vi "Load Production his.vi"(8 "error in (no error)":errorcluster, 9 "Error info (end)":timestamp=timestamp(3727674196.4539065 s since 1904-01-01) format="%<%Y/%m/%d>T", 10 "Error info (start)":timestamp=timestamp(3727674196.4539065 s since 1904-01-01) format="%<%Y/%m/%d>T", 11 "DBlink":string="Driver={ODBC Driver 17 for SQL Server};Server=localhost\\SQLEXPRESS;Database=YDXB01;UID=labview;PWD=123456789") -> (0 "error out":errorcluster, 1 "production_report":T1(array[cluster])=[{"id"=13, "time_supply"="2022/2/14 ¤U¤È 06:05:43", "time_spout"="", "product_num"="F509", "barcode"="400010509", "box"="B", "quality"="NG", "section_time"=0, "total_time"=0}, {"id"=14, "time_supply"="2022/2/14 ¤U¤È 06:05:44", "time_spout"="", "product_num"="F509", "barcode"="400010509", "box"="B", "quality"="NG", "section_time"=0, "total_time"=0}, {"id"=15, "time_supply"="2022/2/14 ¤U¤È 06:05:45", "time_spout"="", "product_num"="F509", "barcode"="400010509", "box"="B", "quality"="NG", "section_time"=0, "total_time"=0}, {"id"=16, "time_supply"="2022/2/14 ¤U¤È 06:05:46", "time_spout"="", "product_num"="F509", "barcode"="400010509", "box"="B", "quality"="NG", "section_time"=0, "total_time"=0}, {"id"=17, "time_supply"="2022/2/14 ¤U¤È 06:05:47", "time_spout"="", "product_num"="F509", "barcode"="400010509", "box"="B", "quality"="NG", "section_time"=0, "total_time"=0}, {"id"=18, "time_supply"="2022/2/14 ¤U¤È 06:05:48", "time_spout"="", "product_num"="F509", "barcode"="400010509", "box"="B", "quality"="NG", "section_time"=0, "total_time"=0}, {"id"=19, "time_supply"="2022/2/14 ¤U¤È 06:05:49", "time_spout"="2022/2/14 ¤U¤È 06:29:45", "product_num"="F509", "barcode"="400010509", "box"="B", "quality"="OK", "section_time"=1290, "total_time"=1436}, {"id"=20, "time_supply"="2022/2/14 ¤U¤È 06:33:46", "time_spout"="", "product_num"="F509", "barcode"="400010509", "box"="B", "quality"="NG", "section_time"=0, "total_time"=0}, {"id"=21, "time_supply"="2022/2/14 ¤U¤È 06:36:11", "time_spout"="2022/2/14 ¤U¤È 06:37:43", "product_num"="F509", "barcode"="400010509", "box"="B", "quality"="OK", "section_time"=2124, "total_time"=92}, {"id"=22, "time_supply"="2022/2/14 ¤U¤È 06:38:07", "time_spout"="", "product_num"="F509", "barcode"="400010509", "box"="B", "quality"="NG", "section_time"=0, "total_time"=0}, {"id"=23, "time_supply"="2022/2/14 ¤U¤È 06:39:35", "time_spout"="2022/2/14 ¤U¤È 06:39:42", "product_num"="F509", "barcode"="400010509", "box"="B", "quality"="OK", "section_time"=2, "total_time"=7}, {"id"=24, "time_supply"="2022/2/14 ¤U¤È 06:39:42", "time_spout"="2022/2/14 ¤U¤È 06:39:50", "product_num"="S504", "barcode"="400010504", "box"="A", "quality"="OK", "section_time"=2, "total_time"=8}, {"id"=25, "time_supply"="2022/2/14 ¤U¤È 06:39:50", "time_spout"="2022/2/14 ¤U¤È 06:39:57", "product_num"="F509", "barcode"="400010509", "box"="B", "quality"="OK", "section_time"=2, "total_time"=7}, {"id"=26, "time_supply"="2022/2/14 ¤U¤È 06:39:57", "time_spout"="2022/2/14 ¤U¤È 06:40:04", "product_num"="F509", "barcode"="400010509", "box"="B", "quality"="OK", "section_time"=2, "total_time"=7}, {"id"=27, "time_supply"="2022/2/14 ¤U¤È 06:40:04", "time_spout"="2022/2/14 ¤U¤È 06:40:14", "product_num"="S504", "barcode"="400010504", "box"="A", "quality"="OK", "section_time"=2, "total_time"=10}, {"id"=28, "time_supply"="2022/2/14 ¤U¤È 06:40:14", "time_spout"="2022/2/14 ¤U¤È 06:40:21", "product_num"="S504", "barcode"="400010504", "box"="A", "quality"="OK", "section_time"=2, "total_time"=7}, {"id"=29, "time_supply"="2022/2/14 ¤U¤È 06:40:21", "time_spout"="2022/2/14 ¤U¤È 06:40:29", "product_num"="S504", "barcode"="400010504", "box"="A", "quality"="OK", "section_time"=2, "total_time"=8}, {"id"=30, "time_supply"="2022/2/14 ¤U¤È 06:40:29", "time_spout"="2022/2/14 ¤U¤È 06:40:36", "product_num"="S504", "barcode"="400010504", "box"="A", "quality"="OK", "section_time"=1, "total_time"=7}, {"id"=31, "time_supply"="2022/2/14 ¤U¤È 06:40:36", "time_spout"="2022/2/14 ¤U¤È 06:40:42", "product_num"="F509", "barcode"="400010509", "box"="B", "quality"="OK", "section_time"=1, "total_time"=6}, {"id"=32, "time_supply"="2022/2/14 ¤U¤È 06:40:42", "time_spout"="2022/2/14 ¤U¤È 06:40:51", "product_num"="S504", "barcode"="400010504", "box"="A", "quality"="OK", "section_time"=2, "total_time"=9}, {"id"=33, "time_supply"="2022/2/14 ¤U¤È 06:40:51", "time_spout"="2022/2/14 ¤U¤È 06:40:57", "product_num"="S504", "barcode"="400010504", "box"="A", "quality"="OK", "section_time"=1, "total_time"=6}, {"id"=34, "time_supply"="2022/2/14 ¤U¤È 06:40:57", "time_spout"="2022/2/14 ¤U¤È 06:41:03", "product_num"="F509", "barcode"="400010509", "box"="B", "quality"="OK", "section_time"=1, "total_time"=6}, {"id"=35, "time_supply"="2022/2/14 ¤U¤È 06:41:03", "time_spout"="2022/2/14 ¤U¤È 06:41:11", "product_num"="S504", "barcode"="400010504", "box"="A", "quality"="OK", "section_time"=1, "total_time"=8}, {"id"=36, "time_supply"="2022/2/14 ¤U¤È 06:41:11", "time_spout"="2022/2/14 ¤U¤È 06:41:18", "product_num"="S504", "barcode"="400010504", "box"="A", "quality"="OK", "section_time"=2, "total_time"=7}, {"id"=37, "time_supply"="2022/2/14 ¤U¤È 06:41:18", "time_spout"="2022/2/14 ¤U¤È 06:41:25", "product_num"="F509", "barcode"="400010509", "box"="B", "quality"="OK", "section_time"=1, "total_time"=7}, {"id"=38, "time_supply"="2022/2/14 ¤U¤È 06:41:25", "time_spout"="2022/2/14 ¤U¤È 06:41:35", "product_num"="F509", "barcode"="400010509", "box"="B", "quality"="OK", "section_time"=2, "total_time"=10}, {"id"=39, "time_supply"="2022/2/14 ¤U¤È 06:41:35", "time_spout"="2022/2/14 ¤U¤È 06:41:43", "product_num"="S504", "barcode"="400010504", "box"="A", "quality"="OK", "section_time"=2, "total_time"=8}, {"id"=40, "time_supply"="2022/2/14 ¤U¤È 06:41:43", "time_spout"="2022/2/14 ¤U¤È 06:41:49", "product_num"="F509", "barcode"="400010509", "box"="B", "quality"="OK", "section_time"=1, "total_time"=6}, {"id"=41, "time_supply"="2022/2/14 ¤U¤È 06:41:49", "time_spout"="2022/2/14 ¤U¤È 06:41:58", "product_num"="F509", "barcode"="400010509", "box"="B", "quality"="OK", "section_time"=2, "total_time"=9}, {"id"=42, "time_supply"="2022/2/14 ¤U¤È 06:41:58", "time_spout"="2022/2/14 ¤U¤È 06:42:08", "product_num"="S504", "barcode"="400010504", "box"="A", "quality"="OK", "section_time"=2, "total_time"=10}, {"id"=43, "time_supply"="2022/2/14 ¤U¤È 06:42:08", "time_spout"="2022/2/14 ¤U¤È 06:42:16", "product_num"="F509", "barcode"="400010509", "box"="B", "quality"="OK", "section_time"=1, "total_time"=8}, {"id"=44, "time_supply"="2022/2/14 ¤U¤È 06:42:16", "time_spout"="2022/2/14 ¤U¤È 06:42:21", "product_num"="S504", "barcode"="400010504", "box"="A", "quality"="OK", "section_time"=1, "total_time"=5}, {"id"=45, "time_supply"="2022/2/14 ¤U¤È 06:42:21", "time_spout"="2022/2/14 ¤U¤È 06:42:30", "product_num"="S504", "barcode"="400010504", "box"="A", "quality"="OK", "section_time"=1, "total_time"=9}, {"id"=46, "time_supply"="2022/2/14 ¤U¤È 06:42:30", "time_spout"="2022/2/14 ¤U¤È 06:42:39", "product_num"="F509", "barcode"="400010509", "box"="B", "quality"="OK", "section_time"=2, "total_time"=9}, {"id"=47, "time_supply"="2022/2/14 ¤U¤È 06:42:39", "time_spout"="2022/2/14 ¤U¤È 06:42:47", "product_num"="S504", "barcode"="400010504", "box"="A", "quality"="OK", "section_time"=2, "total_time"=8}, {"id"=48, "time_supply"="2022/2/14 ¤U¤È 06:42:47", "time_spout"="2022/2/14 ¤U¤È 06:42:54", "product_num"="S504", "barcode"="400010504", "box"="A", "quality"="OK", "section_time"=2, "total_time"=7}, {"id"=49, "time_supply"="2022/2/14 ¤U¤È 06:42:54", "time_spout"="2022/2/14 ¤U¤È 06:43:01", "product_num"="S504", "barcode"="400010504", "box"="A", "quality"="OK", "section_time"=2, "total_time"=7}, {"id"=50, "time_supply"="2022/2/14 ¤U¤È 06:43:01", "time_spout"="2022/2/14 ¤U¤È 06:43:09", "product_num"="F509", "barcode"="400010509", "box"="B", "quality"="OK", "section_time"=2, "total_time"=8}, {"id"=51, "time_supply"="2022/2/14 ¤U¤È 06:43:09", "time_spout"="2022/2/14 ¤U¤È 06:43:16", "product_num"="S504", "barcode"="400010504", "box"="A", "quality"="OK", "section_time"=1, "total_time"=7}, {"id"=52, "time_supply"="2022/2/14 ¤U¤È 06:43:16", "time_spout"="2022/2/14 ¤U¤È 06:43:21", "product_num"="F509", "barcode"="400010509", "box"="B", "quality"="OK", "section_time"=1, "total_time"=5}, {"id"=53, "time_supply"="2022/2/14 ¤U¤È 06:43:21", "time_spout"="2022/2/14 ¤U¤È 06:43:28", "product_num"="F509", "barcode"="400010509", "box"="B", "quality"="OK", "section_time"=1, "total_time"=7}, {"id"=54, "time_supply"="2022/2/14 ¤U¤È 06:43:28", "time_spout"="2022/2/14 ¤U¤È 06:43:36", "product_num"="F509", "barcode"="400010509", "box"="B", "quality"="OK", "section_time"=2, "total_time"=8}, {"id"=55, "time_supply"="2022/2/14 ¤U¤È 06:43:36", "time_spout"="2022/2/14 ¤U¤È 06:43:42", "product_num"="S504", "barcode"="400010504", "box"="A", "quality"="OK", "section_time"=1, "total_time"=6}, {"id"=56, "time_supply"="2022/2/14 ¤U¤È 06:43:42", "time_spout"="2022/2/14 ¤U¤È 06:43:51", "product_num"="F509", "barcode"="400010509", "box"="B", "quality"="OK", "section_time"=2, "total_time"=9}, {"id"=57, "time_supply"="2022/2/14 ¤U¤È 06:43:51", "time_spout"="2022/2/14 ¤U¤È 06:43:59", "product_num"="F509", "barcode"="400010509", "box"="B", "quality"="OK", "section_time"=2, "total_time"=8}, {"id"=58, "time_supply"="2022/2/14 ¤U¤È 06:43:59", "time_spout"="2022/2/14 ¤U¤È 06:44:07", "product_num"="S504", "barcode"="400010504", "box"="A", "quality"="OK", "section_time"=1, "total_time"=8}, {"id"=59, "time_supply"="2022/2/14 ¤U¤È 06:44:07", "time_spout"="2022/2/14 ¤U¤È 06:44:13", "product_num"="S504", "barcode"="400010504", "box"="A", "quality"="OK", "section_time"=1, "total_time"=6}, {"id"=60, "time_supply"="2022/2/14 ¤U¤È 06:44:13", "time_spout"="2022/2/14 ¤U¤È 06:44:18", "product_num"="F509", "barcode"="400010509", "box"="B", "quality"="OK", "section_time"=1, "total_time"=5}, {"id"=61, "time_supply"="2022/2/14 ¤U¤È 06:44:18", "time_spout"="2022/2/14 ¤U¤È 06:44:25", "product_num"="F509", "barcode"="400010509", "box"="B", "quality"="OK", "section_time"=1, "total_time"=7}, {"id"=62, "time_supply"="2022/2/14 ¤U¤È 06:44:25", "time_spout"="2022/2/14 ¤U¤È 06:44:32", "product_num"="F509", "barcode"="400010509", "box"="B", "quality"="OK", "section_time"=1, "total_time"=7}, {"id"=63, "time_supply"="2022/2/14 ¤U¤È 06:44:33", "time_spout"="2022/2/14 ¤U¤È 06:44:40", "product_num"="S504", "barcode"="400010504", "box"="A", "quality"="OK", "section_time"=2, "total_time"=7}, {"id"=64, "time_supply"="2022/2/14 ¤U¤È 06:44:40", "time_spout"="2022/2/14 ¤U¤È 06:44:47", "product_num"="S504", "barcode"="400010504", "box"="A", "quality"="OK", "section_time"=1, "total_time"=7}, {"id"=65, "time_supply"="2022/2/14 ¤U¤È 06:44:47", "time_spout"="2022/2/14 ¤U¤È 06:44:54", "product_num"="F509", "barcode"="400010509", "box"="B", "quality"="OK", "section_time"=1, "total_time"=7}, {"id"=66, "time_supply"="2022/2/14 ¤U¤È 06:44:54", "time_spout"="2022/2/14 ¤U¤È 06:45:02", "product_num"="F509", "barcode"="400010509", "box"="B", "quality"="OK", "section_time"=1, "total_time"=8}, {"id"=67, "time_supply"="2022/2/14 ¤U¤È 06:45:02", "time_spout"="2022/2/14 ¤U¤È 06:45:08", "product_num"="S504", "barcode"="400010504", "box"="A", "quality"="OK", "section_time"=1, "total_time"=6}, {"id"=68, "time_supply"="2022/2/14 ¤U¤È 06:45:08", "time_spout"="2022/2/14 ¤U¤È 06:45:13", "product_num"="F509", "barcode"="400010509", "box"="B", "quality"="OK", "section_time"=1, "total_time"=5}, {"id"=69, "time_supply"="2022/2/14 ¤U¤È 06:45:13", "time_spout"="2022/2/14 ¤U¤È 06:45:19", "product_num"="F509", "barcode"="400010509", "box"="B", "quality"="OK", "section_time"=1, "total_time"=6}, {"id"=70, "time_supply"="2022/2/14 ¤U¤È 06:45:19", "time_spout"="2022/2/14 ¤U¤È 06:45:25", "product_num"="S504", "barcode"="400010504", "box"="A", "quality"="OK", "section_time"=1, "total_time"=6}, {"id"=71, "time_supply"="2022/2/14 ¤U¤È 06:45:25", "time_spout"="2022/2/14 ¤U¤È 06:45:35", "product_num"="S504", "barcode"="400010504", "box"="A", "quality"="OK", "section_time"=2, "total_time"=10}, {"id"=72, "time_supply"="2022/2/14 ¤U¤È 06:45:35", "time_spout"="2022/2/14 ¤U¤È 06:45:41", "product_num"="S504", "barcode"="400010504", "box"="A", "quality"="OK", "section_time"=1, "total_time"=6}, {"id"=73, "time_supply"="2022/2/14 ¤U¤È 06:45:41", "time_spout"="2022/2/14 ¤U¤È 06:45:49", "product_num"="F509", "barcode"="400010509", "box"="B", "quality"="OK", "section_time"=1, "total_time"=8}, {"id"=74, "time_supply"="2022/2/14 ¤U¤È 06:45:49", "time_spout"="2022/2/14 ¤U¤È 06:45:55", "product_num"="F509", "barcode"="400010509", "box"="B", "quality"="OK", "section_time"=1, "total_time"=6}, {"id"=75, "time_supply"="2022/2/14 ¤U¤È 06:45:55", "time_spout"="2022/2/14 ¤U¤È 06:46:02", "product_num"="F509", "barcode"="400010509", "box"="B", "quality"="OK", "section_time"=1, "total_time"=7}, {"id"=76, "time_supply"="2022/2/14 ¤U¤È 06:46:02", "time_spout"="2022/2/14 ¤U¤È 06:46:08", "product_num"="S504", "barcode"="400010504", "box"="A", "quality"="OK", "section_time"=1, "total_time"=6}, {"id"=77, "time_supply"="2022/2/14 ¤U¤È 06:46:08", "time_spout"="2022/2/14 ¤U¤È 06:46:13", "product_num"="F509", "barcode"="400010509", "box"="B", "quality"="OK", "section_time"=1, "total_time"=5}, {"id"=78, "time_supply"="2022/2/14 ¤U¤È 06:46:13", "time_spout"="2022/2/14 ¤U¤È 06:46:21", "product_num"="F509", "barcode"="400010509", "box"="B", "quality"="OK", "section_time"=1, "total_time"=8}, {"id"=79, "time_supply"="2022/2/14 ¤U¤È 06:46:21", "time_spout"="2022/2/14 ¤U¤È 06:46:28", "product_num"="S504", "barcode"="400010504", "box"="A", "quality"="OK", "section_time"=1, "total_time"=7}, {"id"=80, "time_supply"="2022/2/14 ¤U¤È 06:46:28", "time_spout"="2022/2/14 ¤U¤È 06:46:35", "product_num"="F509", "barcode"="400010509", "box"="B", "quality"="OK", "section_time"=2, "total_time"=7}, {"id"=81, "time_supply"="2022/2/14 ¤U¤È 06:46:35", "time_spout"="2022/2/14 ¤U¤È 06:46:45", "product_num"="F509", "barcode"="400010509", "box"="B", "quality"="OK", "section_time"=2, "total_time"=10}, {"id"=82, "time_supply"="2022/2/14 ¤U¤È 06:46:45", "time_spout"="2022/2/14 ¤U¤È 06:46:54", "product_num"="S504", "barcode"="400010504", "box"="A", "quality"="OK", "section_time"=2, "total_time"=9}, {"id"=83, "time_supply"="2022/2/14 ¤U¤È 06:46:54", "time_spout"="2022/2/14 ¤U¤È 06:47:03", "product_num"="S504", "barcode"="400010504", "box"="A", "quality"="OK", "section_time"=2, "total_time"=9}, {"id"=84, "time_supply"="2022/2/14 ¤U¤È 06:47:03", "time_spout"="2022/2/14 ¤U¤È 06:47:13", "product_num"="F509", "barcode"="400010509", "box"="B", "quality"="OK", "section_time"=2, "total_time"=10}, {"id"=85, "time_supply"="2022/2/14 ¤U¤È 06:47:13", "time_spout"="2022/2/14 ¤U¤È 06:47:21", "product_num"="F509", "barcode"="400010509", "box"="B", "quality"="OK", "section_time"=1, "total_time"=8}, {"id"=86, "time_supply"="2022/2/14 ¤U¤È 06:47:21", "time_spout"="2022/2/14 ¤U¤È 06:47:30", "product_num"="F509", "barcode"="400010509", "box"="B", "quality"="OK", "section_time"=2, "total_time"=9}, {"id"=87, "time_supply"="2022/2/14 ¤U¤È 06:47:30", "time_spout"="2022/2/14 ¤U¤È 06:47:39", "product_num"="S504", "barcode"="400010504", "box"="A", "quality"="OK", "section_time"=1, "total_time"=9}, {"id"=88, "time_supply"="2022/2/14 ¤U¤È 06:47:39", "time_spout"="2022/2/14 ¤U¤È 06:47:44", "product_num"="F509", "barcode"="400010509", "box"="B", "quality"="OK", "section_time"=1, "total_time"=5}, {"id"=89, "time_supply"="2022/2/14 ¤U¤È 06:47:44", "time_spout"="2022/2/14 ¤U¤È 06:47:51", "product_num"="F509", "barcode"="400010509", "box"="B", "quality"="OK", "section_time"=1, "total_time"=7}, {"id"=90, "time_supply"="2022/2/14 ¤U¤È 06:47:51", "time_spout"="2022/2/14 ¤U¤È 06:47:59", "product_num"="F509", "barcode"="400010509", "box"="B", "quality"="OK", "section_time"=2, "total_time"=8}, {"id"=91, "time_supply"="2022/2/14 ¤U¤È 06:47:59", "time_spout"="2022/2/14 ¤U¤È 06:48:05", "product_num"="F509", "barcode"="400010509", "box"="B", "quality"="OK", "section_time"=2, "total_time"=6}, {"id"=92, "time_supply"="2022/2/14 ¤U¤È 06:48:05", "time_spout"="2022/2/14 ¤U¤È 06:48:15", "product_num"="S504", "barcode"="400010504", "box"="A", "quality"="OK", "section_time"=2, "total_time"=10}, {"id"=93, "time_supply"="2022/2/14 ¤U¤È 06:48:15", "time_spout"="2022/2/14 ¤U¤È 06:48:21", "product_num"="S504", "barcode"="400010504", "box"="A", "quality"="OK", "section_time"=1, "total_time"=6}, {"id"=94, "time_supply"="2022/2/14 ¤U¤È 06:48:21", "time_spout"="2022/2/14 ¤U¤È 06:48:28", "product_num"="S504", "barcode"="400010504", "box"="A", "quality"="OK", "section_time"=2, "total_time"=7}, {"id"=95, "time_supply"="2022/2/14 ¤U¤È 06:48:28", "time_spout"="2022/2/14 ¤U¤È 06:48:35", "product_num"="S504", "barcode"="400010504", "box"="A", "quality"="OK", "section_time"=2, "total_time"=7}, {"id"=96, "time_supply"="2022/2/14 ¤U¤È 06:48:35", "time_spout"="2022/2/14 ¤U¤È 06:48:44", "product_num"="S504", "barcode"="400010504", "box"="A", "quality"="OK", "section_time"=2, "total_time"=9}, {"id"=97, "time_supply"="2022/2/14 ¤U¤È 06:48:44", "time_spout"="2022/2/14 ¤U¤È 06:48:52", "product_num"="F509", "barcode"="400010509", "box"="B", "quality"="OK", "section_time"=1, "total_time"=8}, {"id"=98, "time_supply"="2022/2/14 ¤U¤È 06:48:52", "time_spout"="2022/2/14 ¤U¤È 06:49:00", "product_num"="S504", "barcode"="400010504", "box"="A", "quality"="OK", "section_time"=1, "total_time"=8}, {"id"=99, "time_supply"="2022/2/14 ¤U¤È 06:49:00", "time_spout"="2022/2/14 ¤U¤È 06:49:08", "product_num"="F509", "barcode"="400010509", "box"="B", "quality"="OK", "section_time"=2, "total_time"=8}, {"id"=100, "time_supply"="2022/2/14 ¤U¤È 06:49:08", "time_spout"="2022/2/14 ¤U¤È 06:49:17", "product_num"="F509", "barcode"="400010509", "box"="B", "quality"="OK", "section_time"=2, "total_time"=9}, {"id"=101, "time_supply"="2022/2/14 ¤U¤È 06:49:17", "time_spout"="2022/2/14 ¤U¤È 06:49:25", "product_num"="S504", "barcode"="400010504", "box"="A", "quality"="OK", "section_time"=2, "total_time"=8}, {"id"=102, "time_supply"="2022/2/14 ¤U¤È 06:49:25", "time_spout"="2022/2/14 ¤U¤È 06:49:33", "product_num"="S504", "barcode"="400010504", "box"="A", "quality"="OK", "section_time"=2, "total_time"=8}, {"id"=103, "time_supply"="2022/2/14 ¤U¤È 06:49:33", "time_spout"="2022/2/14 ¤U¤È 06:49:43", "product_num"="F509", "barcode"="400010509", "box"="B", "quality"="OK", "section_time"=2, "total_time"=10}, {"id"=104, "time_supply"="2022/2/14 ¤U¤È 06:49:43", "time_spout"="2022/2/14 ¤U¤È 06:49:52", "product_num"="S504", "barcode"="400010504", "box"="A", "quality"="OK", "section_time"=2, "total_time"=9}, {"id"=105, "time_supply"="2022/2/14 ¤U¤È 06:49:52", "time_spout"="2022/2/14 ¤U¤È 06:50:00", "product_num"="S504", "barcode"="400010504", "box"="A", "quality"="OK", "section_time"=1, "total_time"=8}, {"id"=106, "time_supply"="2022/2/14 ¤U¤È 06:50:00", "time_spout"="2022/2/14 ¤U¤È 06:50:08", "product_num"="S504", "barcode"="400010504", "box"="A", "quality"="OK", "section_time"=2, "total_time"=8}, {"id"=107, "time_supply"="2022/2/14 ¤U¤È 06:50:08", "time_spout"="2022/2/14 ¤U¤È 06:50:13", "product_num"="F509", "barcode"="400010509", "box"="B", "quality"="OK", "section_time"=1, "total_time"=5}, {"id"=108, "time_supply"="2022/2/14 ¤U¤È 06:50:13", "time_spout"="2022/2/14 ¤U¤È 06:50:23", "product_num"="F509", "barcode"="400010509", "box"="B", "quality"="OK", "section_time"=2, "total_time"=10}, {"id"=109, "time_supply"="2022/2/14 ¤U¤È 06:50:23", "time_spout"="2022/2/14 ¤U¤È 06:50:32", "product_num"="F509", "barcode"="400010509", "box"="B", "quality"="OK", "section_time"=2, "total_time"=9}, {"id"=110, "time_supply"="2022/2/14 ¤U¤È 06:50:32", "time_spout"="2022/2/14 ¤U¤È 06:50:41", "product_num"="S504", "barcode"="400010504", "box"="A", "quality"="OK", "section_time"=2, "total_time"=9}, {"id"=111, "time_supply"="2022/2/14 ¤U¤È 06:50:41", "time_spout"="", "product_num"="F509", "barcode"="400010509", "box"="B", "quality"="NG", "section_time"=0, "total_time"=0}, {"id"=112, "time_supply"="2022/2/14 ¤U¤È 06:51:48", "time_spout"="2022/2/14 ¤U¤È 06:51:55", "product_num"="F509", "barcode"="400010509", "box"="B", "quality"="OK", "section_time"=1, "total_time"=7}, {"id"=113, "time_supply"="2022/2/14 ¤U¤È 06:51:55", "time_spout"="2022/2/14 ¤U¤È 06:52:04", "product_num"="F509", "barcode"="400010509", "box"="B", "quality"="OK", "section_time"=2, "total_time"=9}, {"id"=114, "time_supply"="2022/2/14 ¤U¤È 06:52:04", "time_spout"="2022/2/14 ¤U¤È 06:52:10", "product_num"="S504", "barcode"="400010504", "box"="A", "quality"="OK", "section_time"=1, "total_time"=6}, {"id"=115, "time_supply"="2022/2/14 ¤U¤È 06:52:10", "time_spout"="", "product_num"="S504", "barcode"="400010504", "box"="A", "quality"="NG", "section_time"=0, "total_time"=0}, {"id"=116, "time_supply"="2022/2/14 ¤U¤È 06:52:17", "time_spout"="2022/2/14 ¤U¤È 06:52:27", "product_num"="F509", "barcode"="400010509", "box"="B", "quality"="OK", "section_time"=2, "total_time"=10}, {"id"=117, "time_supply"="2022/2/14 ¤U¤È 06:52:27", "time_spout"="", "product_num"="S504", "barcode"="400010504", "box"="A", "quality"="NG", "section_time"=0, "total_time"=0}, {"id"=118, "time_supply"="2022/2/14 ¤U¤È 06:52:35", "time_spout"="2022/2/14 ¤U¤È 06:52:41", "product_num"="S504", "barcode"="400010504", "box"="A", "quality"="OK", "section_time"=1, "total_time"=6}, {"id"=119, "time_supply"="2022/2/14 ¤U¤È 06:52:41", "time_spout"="2022/2/14 ¤U¤È 06:52:46", "product_num"="S504", "barcode"="400010504", "box"="A", "quality"="OK", "section_time"=1, "total_time"=5}, {"id"=120, "time_supply"="2022/2/14 ¤U¤È 06:52:46", "time_spout"="2022/2/14 ¤U¤È 06:52:55", "product_num"="S504", "barcode"="400010504", "box"="A", "quality"="OK", "section_time"=2, "total_time"=9}, {"id"=121, "time_supply"="2022/2/14 ¤U¤È 06:52:55", "time_spout"="2022/2/14 ¤U¤È 06:53:03", "product_num"="S504", "barcode"="400010504", "box"="A", "quality"="OK", "section_time"=1, "total_time"=8}, {"id"=122, "time_supply"="2022/2/14 ¤U¤È 06:53:03", "time_spout"="2022/2/14 ¤U¤È 06:53:09", "product_num"="S504", "barcode"="400010504", "box"="A", "quality"="OK", "section_time"=1, "total_time"=6}, {"id"=123, "time_supply"="2022/2/14 ¤U¤È 06:53:09", "time_spout"="", "product_num"="S504", "barcode"="400010504", "box"="A", "quality"="NG", "section_time"=0, "total_time"=0}, {"id"=124, "time_supply"="2022/2/14 ¤U¤È 06:53:15", "time_spout"="2022/2/14 ¤U¤È 06:53:22", "product_num"="S504", "barcode"="400010504", "box"="A", "quality"="OK", "section_time"=2, "total_time"=7}, {"id"=125, "time_supply"="2022/2/14 ¤U¤È 06:53:22", "time_spout"="", "product_num"="F509", "barcode"="400010509", "box"="B", "quality"="NG", "section_time"=0, "total_time"=0}, {"id"=126, "time_supply"="2022/2/14 ¤U¤È 06:53:30", "time_spout"="2022/2/14 ¤U¤È 06:53:35", "product_num"="S504", "barcode"="400010504", "box"="A", "quality"="OK", "section_time"=1, "total_time"=5}, {"id"=127, "time_supply"="2022/2/14 ¤U¤È 06:53:35", "time_spout"="", "product_num"="S504", "barcode"="400010504", "box"="A", "quality"="NG", "section_time"=0, "total_time"=0}, {"id"=128, "time_supply"="2022/2/14 ¤U¤È 06:53:42", "time_spout"="", "product_num"="F509", "barcode"="400010509", "box"="B", "quality"="NG", "section_time"=0, "total_time"=0}, {"id"=129, "time_supply"="2022/2/14 ¤U¤È 06:53:50", "time_spout"="2022/2/14 ¤U¤È 06:53:59", "product_num"="F509", "barcode"="400010509", "box"="B", "quality"="OK", "section_time"=1, "total_time"=9}, {"id"=130, "time_supply"="2022/2/14 ¤U¤È 06:53:59", "time_spout"="2022/2/14 ¤U¤È 06:54:06", "product_num"="F509", "barcode"="400010509", "box"="B", "quality"="OK", "section_time"=1, "total_time"=7}, {"id"=131, "time_supply"="2022/2/14 ¤U¤È 06:54:06", "time_spout"="2022/2/14 ¤U¤È 06:54:13", "product_num"="F509", "barcode"="400010509", "box"="B", "quality"="OK", "section_time"=2, "total_time"=7}, {"id"=132, "time_supply"="2022/2/14 ¤U¤È 06:54:13", "time_spout"="", "product_num"="S504", "barcode"="400010504", "box"="A", "quality"="NG", "section_time"=0, "total_time"=0}, {"id"=133, "time_supply"="2022/2/14 ¤U¤È 06:54:19", "time_spout"="", "product_num"="S504", "barcode"="400010504", "box"="A", "quality"="NG", "section_time"=0, "total_time"=0}, {"id"=134, "time_supply"="2022/2/14 ¤U¤È 06:54:37", "time_spout"="2022/2/14 ¤U¤È 06:54:43", "product_num"="S504", "barcode"="400010504", "box"="A", "quality"="OK", "section_time"=1, "total_time"=6}, {"id"=135, "time_supply"="2022/2/14 ¤U¤È 06:54:43", "time_spout"="2022/2/14 ¤U¤È 06:54:49", "product_num"="S504", "barcode"="400010504", "box"="A", "quality"="OK", "section_time"=2, "total_time"=6}, {"id"=136, "time_supply"="2022/2/14 ¤U¤È 06:54:49", "time_spout"="2022/2/14 ¤U¤È 06:54:55", "product_num"="F509", "barcode"="400010509", "box"="B", "quality"="OK", "section_time"=1, "total_time"=6}, {"id"=137, "time_supply"="2022/2/14 ¤U¤È 06:54:55", "time_spout"="2022/2/14 ¤U¤È 06:55:05", "product_num"="S504", "barcode"="400010504", "box"="A", "quality"="OK", "section_time"=2, "total_time"=10}, {"id"=138, "time_supply"="2022/2/14 ¤U¤È 06:55:05", "time_spout"="2022/2/14 ¤U¤È 06:55:10", "product_num"="S504", "barcode"="400010504", "box"="A", "quality"="OK", "section_time"=1, "total_time"=5}, {"id"=139, "time_supply"="2022/2/14 ¤U¤È 06:55:10", "time_spout"="2022/2/14 ¤U¤È 06:55:19", "product_num"="S504", "barcode"="400010504", "box"="A", "quality"="OK", "section_time"=2, "total_time"=9}, {"id"=140, "time_supply"="2022/2/14 ¤U¤È 06:55:19", "time_spout"="2022/2/14 ¤U¤È 06:55:27", "product_num"="F509", "barcode"="400010509", "box"="B", "quality"="OK", "section_time"=1, "total_time"=8}, {"id"=141, "time_supply"="2022/2/14 ¤U¤È 06:55:27", "time_spout"="2022/2/14 ¤U¤È 06:55:33", "product_num"="F509", "barcode"="400010509", "box"="B", "quality"="OK", "section_time"=1, "total_time"=6}, {"id"=142, "time_supply"="2022/2/14 ¤U¤È 06:55:33", "time_spout"="2022/2/14 ¤U¤È 06:55:41", "product_num"="F509", "barcode"="400010509", "box"="B", "quality"="OK", "section_time"=1, "total_time"=8}, {"id"=143, "time_supply"="2022/2/14 ¤U¤È 06:55:41", "time_spout"="", "product_num"="S504", "barcode"="400010504", "box"="A", "quality"="NG", "section_time"=0, "total_time"=0}, {"id"=144, "time_supply"="2022/2/14 ¤U¤È 06:55:48", "time_spout"="2022/2/14 ¤U¤È 06:55:56", "product_num"="S504", "barcode"="400010504", "box"="A", "quality"="OK", "section_time"=1, "total_time"=8}, {"id"=145, "time_supply"="2022/2/14 ¤U¤È 06:55:56", "time_spout"="2022/2/14 ¤U¤È 06:56:06", "product_num"="S504", "barcode"="400010504", "box"="A", "quality"="OK", "section_time"=2, "total_time"=10}, {"id"=146, "time_supply"="2022/2/14 ¤U¤È 06:56:06", "time_spout"="2022/2/14 ¤U¤È 06:56:14", "product_num"="F509", "barcode"="400010509", "box"="B", "quality"="OK", "section_time"=1, "total_time"=8}, {"id"=147, "time_supply"="2022/2/14 ¤U¤È 06:56:14", "time_spout"="", "product_num"="S504", "barcode"="400010504", "box"="A", "quality"="NG", "section_time"=0, "total_time"=0}])   [LabVIEW 2019]
uses:
  <vilib>/addons/database/Connection.llb/DB Tools Open Connec (String).vi
  <vilib>/addons/database/_DB Variant To Data/Database Variant To Data.xnode
  <vilib>/addons/database/NI_Database_API.lvlib
panel:
  in  "columns":string[](array[string])=["id", "time_supply", "time_spout", "product_num", "barcode", "box", "quality", "section_time", "total_time"]
  out "concatenated string":string="where create_time between '2022-2-14' AND '2022-2-14 23:59:59'"
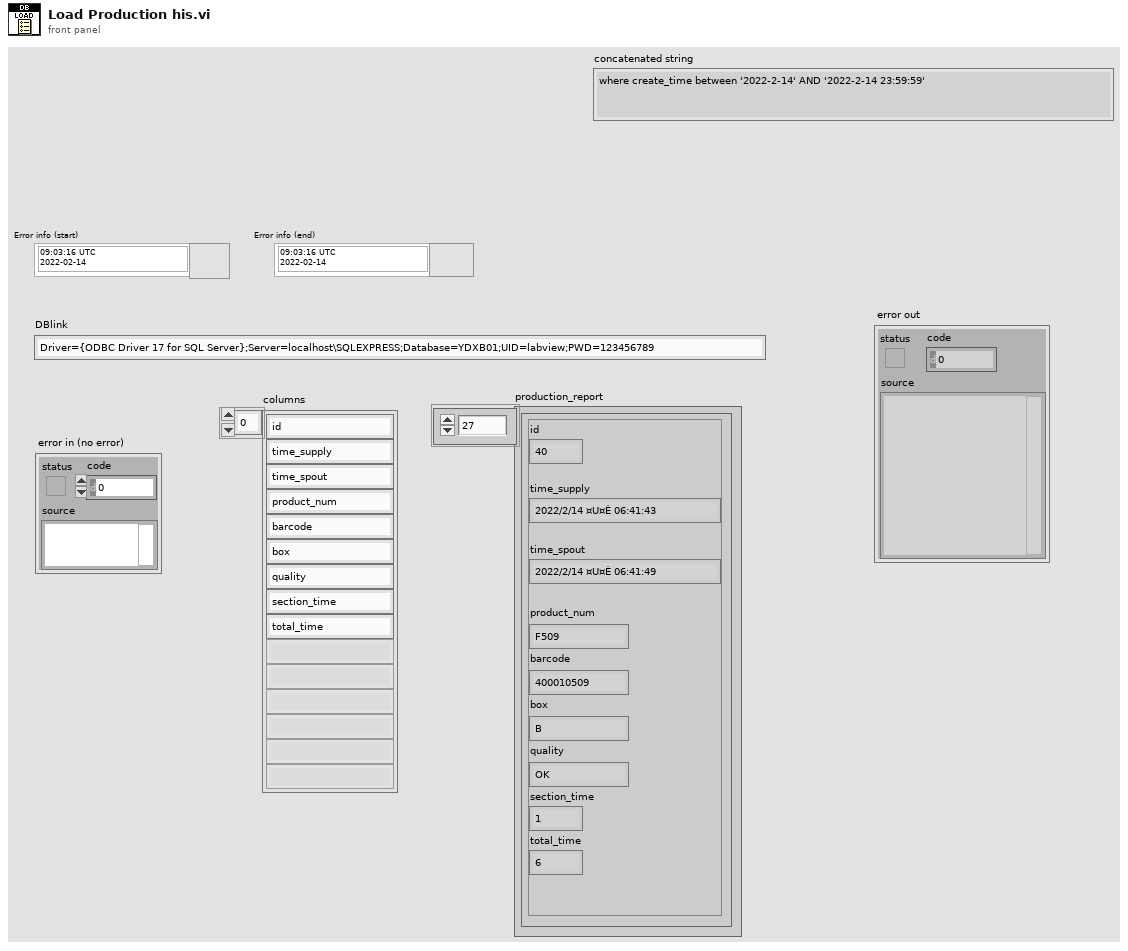
[diagram p1: front panel]
types:
  T1 = cluster{"id":i32, "time_supply":string, "time_spout":string, "product_num":string, "barcode":string, "box":string, "quality":string, "section_time":i32, "total_time":i32}[]
  T2 = typedef "NI_Database_API.lvlib/Conn ObjectReference.ctl" = refnum<k1>
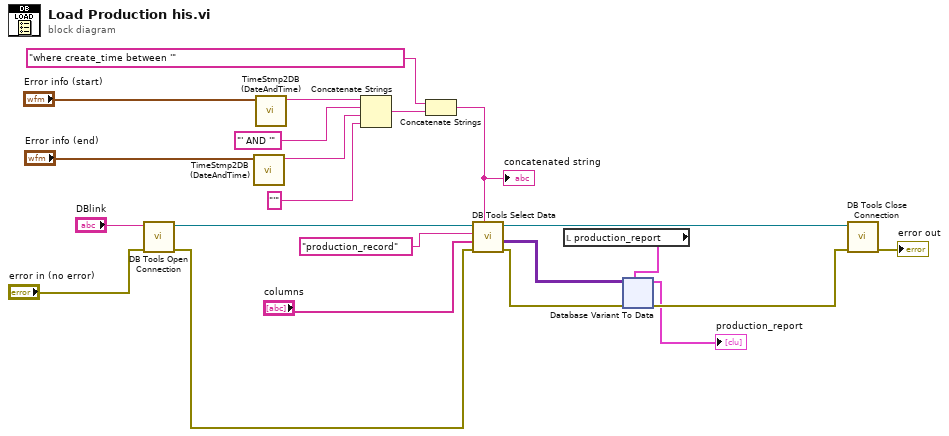
[diagram p0: block diagram]
diagram:
  n1 = call-poly <vilib>:"DB Tools Open Connection.vi"("error in (no error)"="error in (no error)", "connection information"="DBlink") -> ("error out"=w16:errorcluster, "connection reference"=w17:T2)  [unwired: 6 in]
  n2 = call "TimeStmp2DB (DateAndTime).vi"("time_Logout"="Error info (end)") -> ("date/time string"=w1:string)  [unwired: 10 in]
  n3 = call "TimeStmp2DB (DateAndTime).vi"("time_Logout"="Error info (start)") -> ("date/time string"=w3:string)  [unwired: 10 in]
  n4 = Concatenate Strings(w3, "' AND '" ("string"), w1, "'" ("string")) -> (w10:string)
  n5 = Concatenate Strings("where create_time between '" ("format string"), w10) -> (w9:string)
  "concatenated string" <- w9
  n6 = call <vilib>:"DB Tools Select Data.vi"("condition"=w9, "error in (no error)"=w16, "columns"="columns", "table"="production_record", "connection reference"=w17) -> ("error out"=w8:errorcluster, "data"=w22:variant[][], "connection reference out"=w14:T2)  [unwired: 1 in]
  n7 = local read "production_report"() -> (w20:T1)
  n8 = xnode "Database Variant To Data"("database variant"=w22, "error in (no error)"=w8, "type"=w20) -> ("data"=→"production_report":T1, "error out"=w7:errorcluster)
  n9 = call <vilib>:"DB Tools Close Connection.vi"("error in (no error)"=w7, "connection reference"=w14) -> ("error out"=→"error out":errorcluster)  [unwired: 5 in]
